vi "Section07_UpdateUI-01-Enable Start_Disable Stop.vi"(8 "error in (no error)":errorcluster, 11 "QSM_ShiftRegister  in":T1) -> (0 "error out":errorcluster, 3 "QSM_ShiftRegister out":T1)   [LabVIEW 2014, in "GUIUpdateQSM.lvlib"]
uses:
  GUIUpdateQSM.lvlib
  Controls/QSM_ShiftRegister.ctl
  QueueMaintenance/TypeDef/QSMRef_ALL.ctl
  Controls/QSM_Reference.ctl
  Controls/QSM_DataType.ctl
  Controls/QSM_RunStates.ctl
  Queue_TEST/Controls/QSM_Reference.ctl
  Queue_TEST/Controls/QSM_DataType.ctl
  Queue_TEST/Controls/QSM_RunStates.ctl
  Controls/TypeDef_FrontPanelReferences.ctl
  QueueMaintenance/QueueMaintenance.lvlib
  Queue_TEST/TestQSM.lvlib
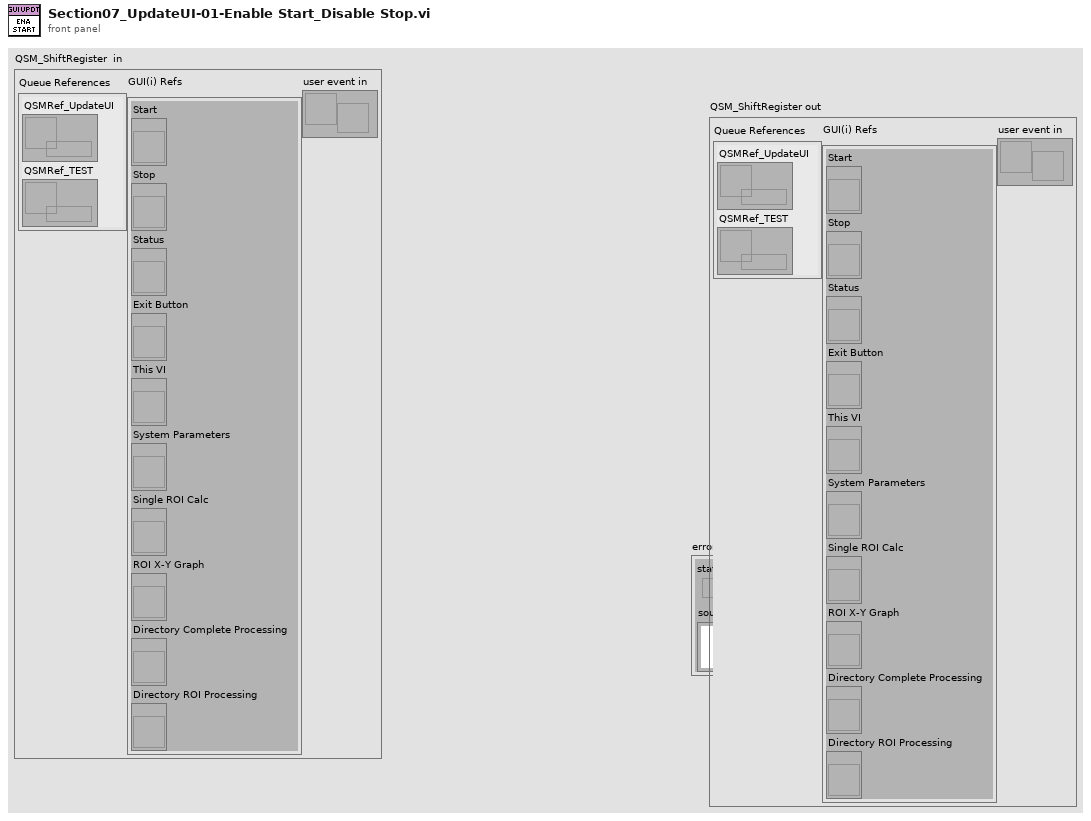
[diagram p1: front panel]
types:
  T1 = typedef "GUIUpdateQSM.lvlib/QSM_ShiftRegister.ctl" = cluster{"Queue References":T2, "GUI(i) Refs":T5, "user event in":refnum<user-event>}
  T2 = typedef "QueueMaintenance.lvlib/QSMRef_ALL.ctl" = cluster{"QSMRef_UpdateUI":T3, "QSMRef_TEST":T4}
  T3 = typedef "GUIUpdateQSM.lvlib/QSM_Reference.ctl" = refnum<queue>
  T4 = typedef "TestQSM.lvlib/QSM_Reference.ctl" = refnum<queue>
  T5 = typedef "GUIUpdateQSM.lvlib/TypeDef_FrontPanelReferences.ctl" = cluster{"Start":refnum<vi>, "Stop":refnum<vi>, "Status":refnum<vi>, "Exit Button":refnum<vi>, "This VI":refnum<vi>, "System Parameters":refnum<vi>, "Single ROI Calc":refnum<vi>, "ROI X-Y Graph":refnum<vi>, "Directory Complete Processing":refnum<vi>, "Directory ROI Processing":refnum<vi>}
  T6 = enum8{"Enabled", "Disabled", "Disabled and Grayed Out"}
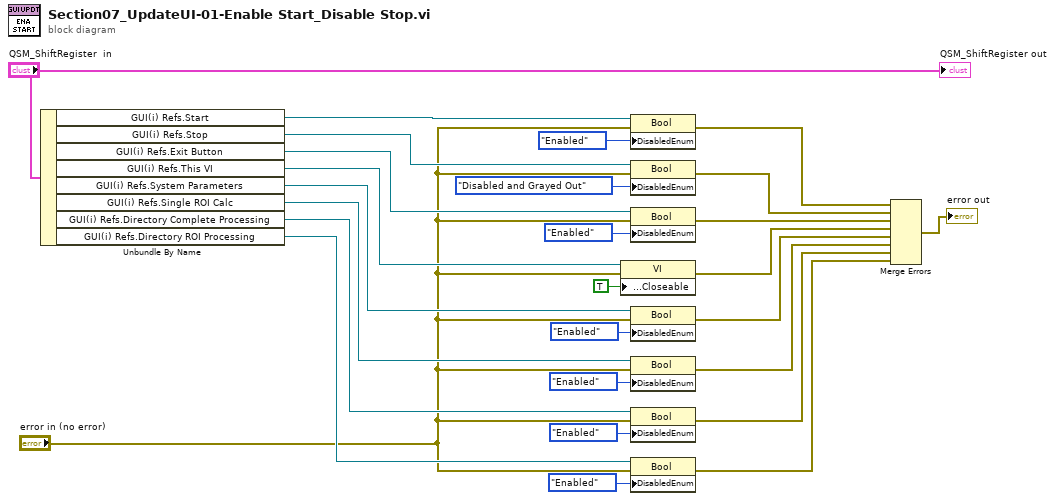
[diagram p0: block diagram]
diagram:
  n1 = Unbundle By Name("QSM_ShiftRegister  in") -> ("GUI(i) Refs.Start"=w26:refnum<vi>, "GUI(i) Refs.Stop"=w21:refnum<vi>, "GUI(i) Refs.Exit Button"=w18:refnum<vi>, "GUI(i) Refs.This VI"=w17:refnum<vi>, "GUI(i) Refs.System Parameters"=w12:refnum<vi>, "GUI(i) Refs.Single ROI Calc"=w9:refnum<vi>, "GUI(i) Refs.Directory Complete Processing"=w5:refnum<vi>, "GUI(i) Refs.Directory ROI Processing"=w4:refnum<vi>)
  n2 = property class="VI"(reference=w17, error in="error in (no error)", "Front Panel.Closeable"=TRUE ("Front Panel Window:Closeable")) -> (error out=w15:errorcluster)  [unwired: 1 out]
  n3 = property class="Bool"(reference=w26, error in="error in (no error)", "DisabledEnum"=T6."Enabled" ("Disabled")) -> (error out=w24:errorcluster)  [unwired: 1 out]
  n4 = property class="Bool"(reference=w21, error in="error in (no error)", "DisabledEnum"=T6."Disabled and Grayed Out" ("Disabled")) -> (error out=w20:errorcluster)  [unwired: 1 out]
  n5 = property class="Bool"(reference=w18, error in="error in (no error)", "DisabledEnum"=T6."Enabled" ("Disabled")) -> (error out=w16:errorcluster)  [unwired: 1 out]
  n6 = property class="Bool"(reference=w12, error in="error in (no error)", "DisabledEnum"=T6."Enabled" ("Disabled")) -> (error out=w11:errorcluster)  [unwired: 1 out]
  n7 = property class="Bool"(reference=w9, error in="error in (no error)", "DisabledEnum"=T6."Enabled" ("Disabled")) -> (error out=w8:errorcluster)  [unwired: 1 out]
  n8 = property class="Bool"(reference=w5, error in="error in (no error)", "DisabledEnum"=T6."Enabled" ("Disabled")) -> (error out=w3:errorcluster)  [unwired: 1 out]
  n9 = property class="Bool"(reference=w4, error in="error in (no error)", "DisabledEnum"=T6."Enabled" ("Disabled")) -> (error out=w2:errorcluster)  [unwired: 1 out]
  n10 = Merge Errors(w24, w20, w16, w15, w11, w8, w3, w2) -> (→"error out":errorcluster)
  "QSM_ShiftRegister out" <- "QSM_ShiftRegister  in"
